vi "PicoInitVisa.vi"(8 "errin":errorcluster, 11 "visain":refnum<visa-resource-name>="COM4") -> (0 "sortie d'erreur":errorcluster caption="errout", 1 "buffer de lecture 2":string, 2 "buffer de lecture":string, 3 "data out":string)   [LabVIEW 2020]
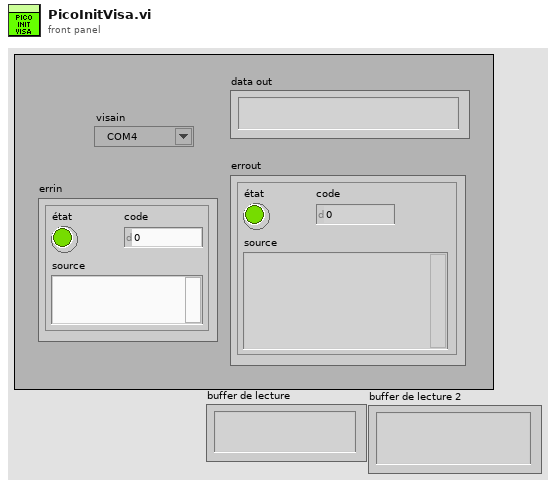
[diagram p1: front panel]
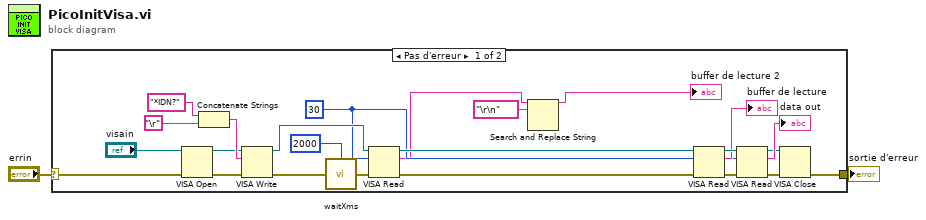
[diagram p0: block diagram]
diagram:
  n1 = case shown="Pas d'erreur" "errin" {
    selector: "errin" -> [w8 w27]
    tunnel: [w15 w27] -> w2
    frame No Error {
      w6 = u32 30 ("nombre d'octets")
      n2 = VISA Open(error in (no error)=w8, VISA resource name="visain") -> (VISA resource name=w11:refnum<visa-resource-name>, error out=w10:errorcluster)  [unwired: 3 in]
      n3 = Concatenate Strings("*IDN?" ("buffer d'écriture"), "\r") -> (w14:string)
      n4 = VISA Write(VISA resource name=w11, write buffer=w14, error in (no error)=w10) -> (VISA resource name out=w9:refnum<visa-resource-name>, error out=w17:errorcluster)  [unwired: 1 out]
      n5 = call "waitXms.vi"("attente (ms)"=u32 2000, "errin"=w17) -> ("errout"=w16:errorcluster)  [unwired: 13 in]
      n6 = VISA Read(VISA resource name=w9, byte count=w6, error in (no error)=w16) -> (VISA resource name out=w20:refnum<visa-resource-name>, read buffer=w5:string, error out=w21:errorcluster)  [unwired: 1 out]
      n7 = Search and Replace String(input string=w5, search string="\r\n" ("chaîne recherchée")) -> (result string=→"buffer de lecture 2":string)  [unwired: 6 in, 3 out]
      n8 = VISA Read(VISA resource name=w20, byte count=w6, error in (no error)=w21) -> (VISA resource name out=w22:refnum<visa-resource-name>, read buffer=→"buffer de lecture":string, error out=w23:errorcluster)  [unwired: 1 out]
      n9 = VISA Read(VISA resource name=w22, byte count=w6, error in (no error)=w23) -> (VISA resource name out=w25:refnum<visa-resource-name>, read buffer=→"data out":string, error out=w24:errorcluster)  [unwired: 1 out]
      n10 = VISA Close(VISA resource name=w25, error in (no error)=w24) -> (error out=w15:errorcluster)
    }
    frame Error {
    }
  }
  "sortie d'erreur" <- w2
